vi "Update Status.vi"(1 "Value":string, 2 "error in (no error)":errorcluster, 6 "States":string, 8 "Str Refnum":refnum<vi>, 10 "Main Step Refnum":refnum<vi>) -> (16 "error out":errorcluster)   [LabVIEW 2014, in "Endigit.lvlib"]
uses:
  Endigit.lvlib
  <vilib>/Utility/error.llb/DialogType.ctl
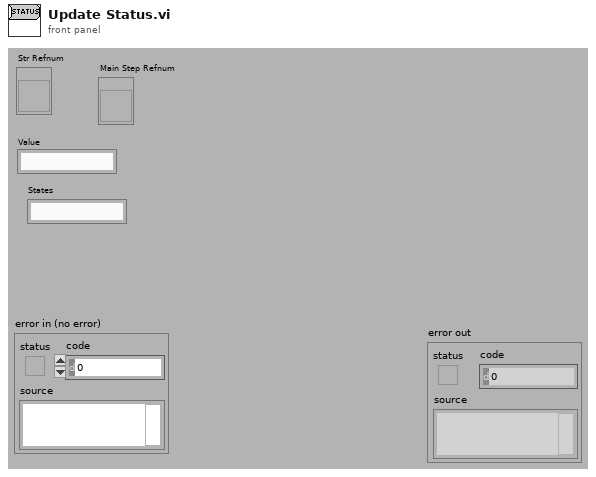
[diagram p1: front panel]
types:
  T1 = typedef "DialogType.ctl" = u16
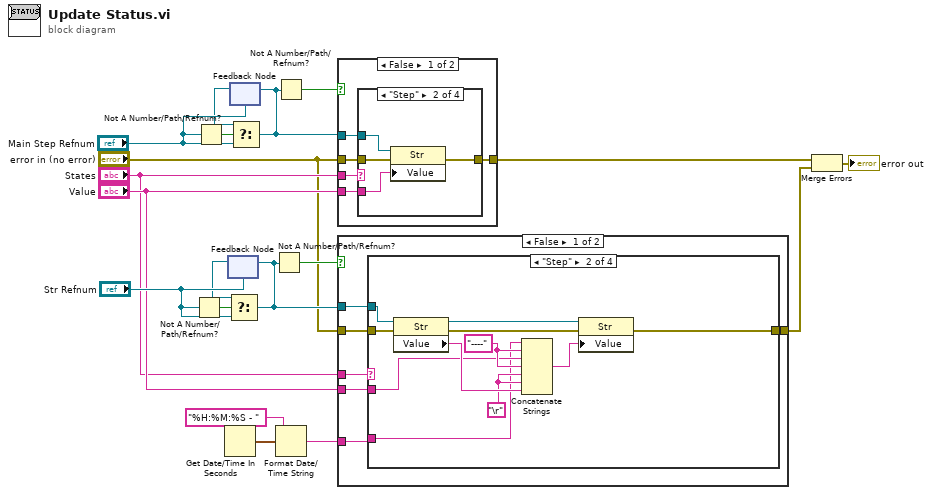
[diagram p0: block diagram]
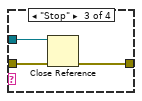
[diagram p3: hidden frame]
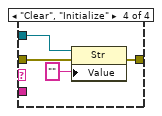
[diagram p4: hidden frame]
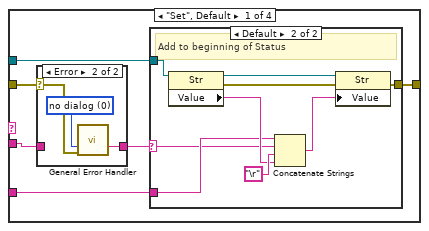
[diagram p6: hidden frame]
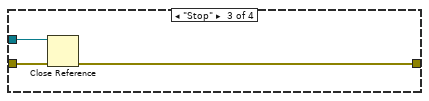
[diagram p9: hidden frame]
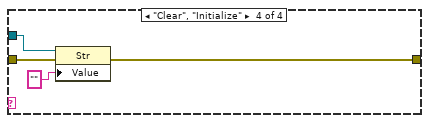
[diagram p10: hidden frame]
diagram:
  n1 = Not A Number/Path/Refnum?(number/path/refnum="Str Refnum") -> (NaN/Path/Refnum?=w14:bool)
  n2 = Not A Number/Path/Refnum?(number/path/refnum="Main Step Refnum") -> (NaN/Path/Refnum?=w4:bool)
  n3 = Get Date/Time In Seconds() -> (seconds since 1Jan1904=w3:timestamp)
  n4 = feedback #1("Str Refnum") -> (w13:refnum<vi>)
  n5 = Select(t=w13, s=w14, f="Str Refnum") -> (s? t:f=w17:refnum<vi>)
  n6 = feedback-in #1(w17) -> ()
  n7 = feedback #2("Main Step Refnum") -> (w5:refnum<vi>)
  n8 = Select(t=w5, s=w4, f="Main Step Refnum") -> (s? t:f=w7:refnum<vi>)
  n9 = feedback-in #2(w7) -> ()
  n10 = Not A Number/Path/Refnum?(number/path/refnum=w17) -> (NaN/Path/Refnum?=w15:bool)
  n11 = Not A Number/Path/Refnum?(number/path/refnum=w7) -> (NaN/Path/Refnum?=w12:bool)
  n12 = Format Date/Time String(time format string (%c)="%H:%M:%S - ", seconds (now)=w3) -> (date/time string=w8:string)  [unwired: 1 in]
  n13 = case shown="False" w12 {
    tunnel: [w24 w37] -> w1
    tunnel: w7 -> [w23 _]
    tunnel: "error in (no error)" -> [w22 w37]
    tunnel: "States" -> [w21 _]
    tunnel: "Value" -> [w20 _]
    frame False {
      n14 = case shown="\"Step\"" w21 {
        tunnel: w20 -> [_ w27 _ _]
        tunnel: w22 -> [w25 w28 w31 w36]
        tunnel: [w25 w26 w30 w35] -> w24
        tunnel: w23 -> [_ w29 w32 w33]
        frame "Set", Default {
        }
        frame "Step" {
          n15 = property class="Str"(reference=w29, error in=w28, "Value"=w27) -> (error out=w26:errorcluster)  [unwired: 1 out]
        }
        frame "Stop" {
          n16 = Close Reference(reference=w32, error in (no error)=w31) -> (error out=w30:errorcluster)
        }
        frame "Clear", "Initialize" {
          n17 = property class="Str"(reference=w33, error in=w36, "Value"="") -> (error out=w35:errorcluster)  [unwired: 1 out]
        }
      }
    }
    frame True {
    }
  }
  n18 = case shown="False" w15 {
    tunnel: w17 -> [w43 _]
    tunnel: w8 -> [w42 _]
    tunnel: "error in (no error)" -> [w41 w81]
    tunnel: "States" -> [w40 _]
    tunnel: "Value" -> [w39 _]
    tunnel: [w38 w81] -> w19
    frame False {
      n19 = case shown="\"Step\"" w40 {
        tunnel: w43 -> [w48 w73 w76 w79]
        tunnel: w39 -> [w46 w66 _ _]
        tunnel: w41 -> [w44 w72 w75 w80]
        tunnel: [w49 w63 w74 w78] -> w38
        tunnel: w42 -> [w47 w65 _ _]
        frame "Set", Default {
          n20 = case shown="Error" w44 {
            selector: w44 -> [_ w62]
            tunnel: [w59 w60] -> w45
            tunnel: w46 -> [w59 _]
            frame No Error {
            }
            frame Error {
              w61 = T1 0 items=["no dialog", "OK message", "continue or stop message", "OK message + warnings", "continue/stop + warnings"] ("type of dialog (OK msg:1)")
              n21 = call <vilib>:"General Error Handler.vi"("type of dialog (OK msg:1)"=w61, "error in (no error)"=w62) -> ("message"=w60:string)  [unwired: 9 in, 4 out]
            }
          }
          n22 = case shown="Default" w45 {
            selector: w45 -> [_ w50]
            tunnel: [_ w58] -> w49
            tunnel: w48 -> [_ w57]
            tunnel: w47 -> [_ w51]
            frame "" {
            }
            frame Default {
              # "Add to beginning of Status"
              n23 = property class="Str"(reference=w57) -> (reference out=w56:refnum<vi>, error out=w55:errorcluster, "Value"=w52:string)  [unwired: 1 in]
              n24 = Concatenate Strings(w51, w50, "\r", w52) -> (w53:string)
              n25 = property class="Str"(reference=w56, error in=w55, "Value"=w53) -> (error out=w58:errorcluster)  [unwired: 1 out]
            }
          }
        }
        frame "Step" {
          w67 = "----" ("string")
          w68 = "\r"
          n26 = property class="Str"(reference=w73, error in=w72) -> (reference out=w71:refnum<vi>, error out=w70:errorcluster, "Value"=w69:string)
          n27 = Concatenate Strings(w65, w67, w66, w67, w68, w68, w69) -> (w64:string)
          n28 = property class="Str"(reference=w71, error in=w70, "Value"=w64) -> (error out=w63:errorcluster)  [unwired: 1 out]
        }
        frame "Stop" {
          n29 = Close Reference(reference=w76, error in (no error)=w75) -> (error out=w74:errorcluster)
        }
        frame "Clear", "Initialize" {
          n30 = property class="Str"(reference=w79, error in=w80, "Value"="") -> (error out=w78:errorcluster)  [unwired: 1 out]
        }
      }
    }
    frame True {
    }
  }
  n31 = Merge Errors(w1, w19) -> (→"error out":errorcluster)
